vi "Connect to NART.vi"(0 "CART TCP Connection In":refnum<k5>, 5 "NART IP Address (localhost)":string="localhost", 7 "NART port (2390)":u32, 11 "error in (no error)":errorcluster) -> (4 "CART TCP Connection Out":refnum<k5>, 15 "error out":errorcluster)   [LabVIEW 2011, in "ART2 Test Panel.lvlib"]
uses:
  ART2 Test Panel.lvlib
  Controls/Connect_device.ctl
panel:
  in  "NART Device/Instance":T1
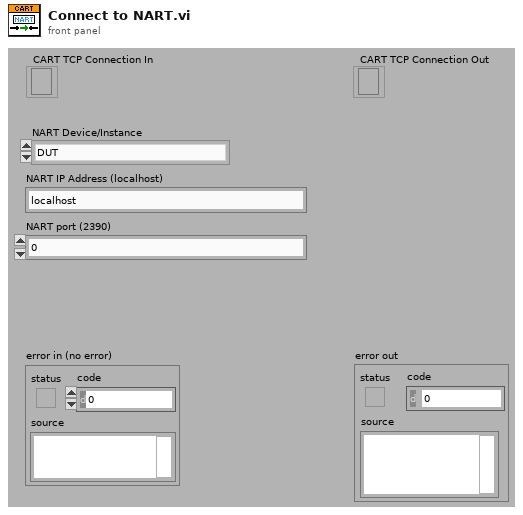
[diagram p1: front panel]
types:
  T1 = typedef "ART2 Test Panel.lvlib/Connect_device.ctl" = enum16{"DUT", "Golden", "Blocker"}
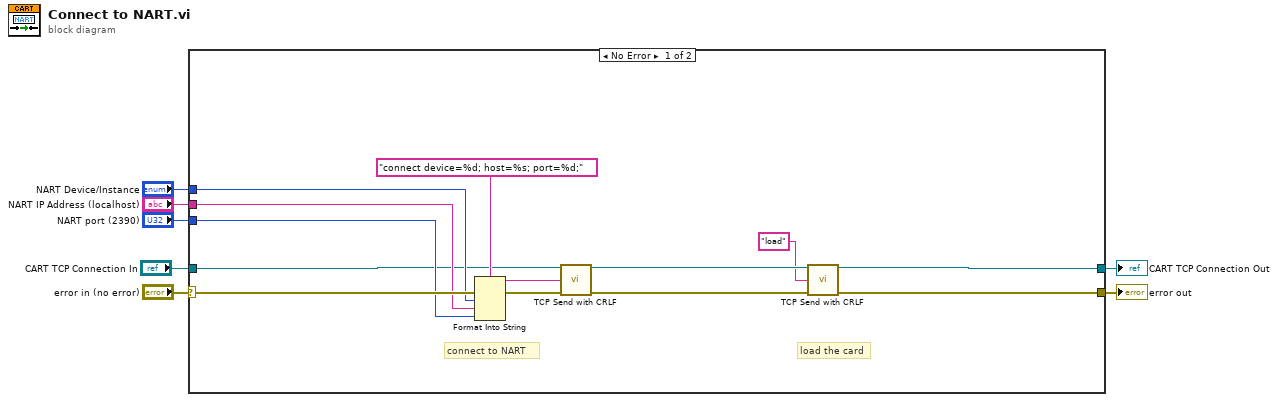
[diagram p0: block diagram]
diagram:
  n1 = case shown="No Error" "error in (no error)" {
    selector: "error in (no error)" -> [w19 w22]
    tunnel: [w10 w22] -> w5
    tunnel: "NART port (2390)" -> [w16 _]
    tunnel: "CART TCP Connection In" -> [w14 w21]
    tunnel: "NART Device/Instance" -> [w18 _]
    tunnel: "NART IP Address (localhost)" -> [w17 _]
    tunnel: [w13 w21] -> w1
    frame No Error {
      # "connect to NART"
      # "load the card"
      n2 = Format Into String(format string="connect device=%d; host=%s; port=%d;", error in=w19, w18, w17, w16) -> (resulting string=w8:string, error out=w15:errorcluster)  [unwired: 1 in]
      n3 = call "TCP Send with CRLF.vi"("CART TCP Connection"=w14, "data in"=w8, "error IO"=w15) -> ("CART TCP Connection Out"=w12:refnum<k5>, "error out"=w11:errorcluster)  [unwired: 11 in]
      n4 = call "TCP Send with CRLF.vi"("CART TCP Connection"=w12, "data in"="load", "error IO"=w11) -> ("CART TCP Connection Out"=w13:refnum<k5>, "error out"=w10:errorcluster)  [unwired: 11 in]
    }
    frame Error {
    }
  }
  "error out" <- w5
  "CART TCP Connection Out" <- w1
